vi "SigProc_subVI smoothBoxcarAvg.vi"(6 "Size":i32=1 min=1 max=100000, 11 "Spectra in":cluster{"X":dbl[], "Y":dbl[]}[](array[cluster])) -> (3 "Spectra out":cluster{"X":dbl[], "Y":dbl[]}[](array[cluster]))   [LabVIEW 2018, in "Sig2MS.lvclass"]
uses:
  Sig2MS.lvclass
  <vilib>/Analysis/baseanly.llb/Mean (DBL).vi
  <vilib>/Analysis/NI_AALBase.lvlib
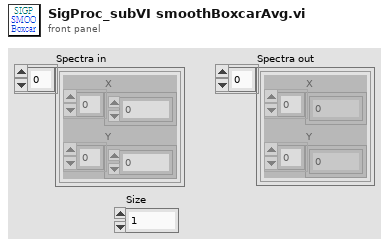
[diagram p1: front panel]
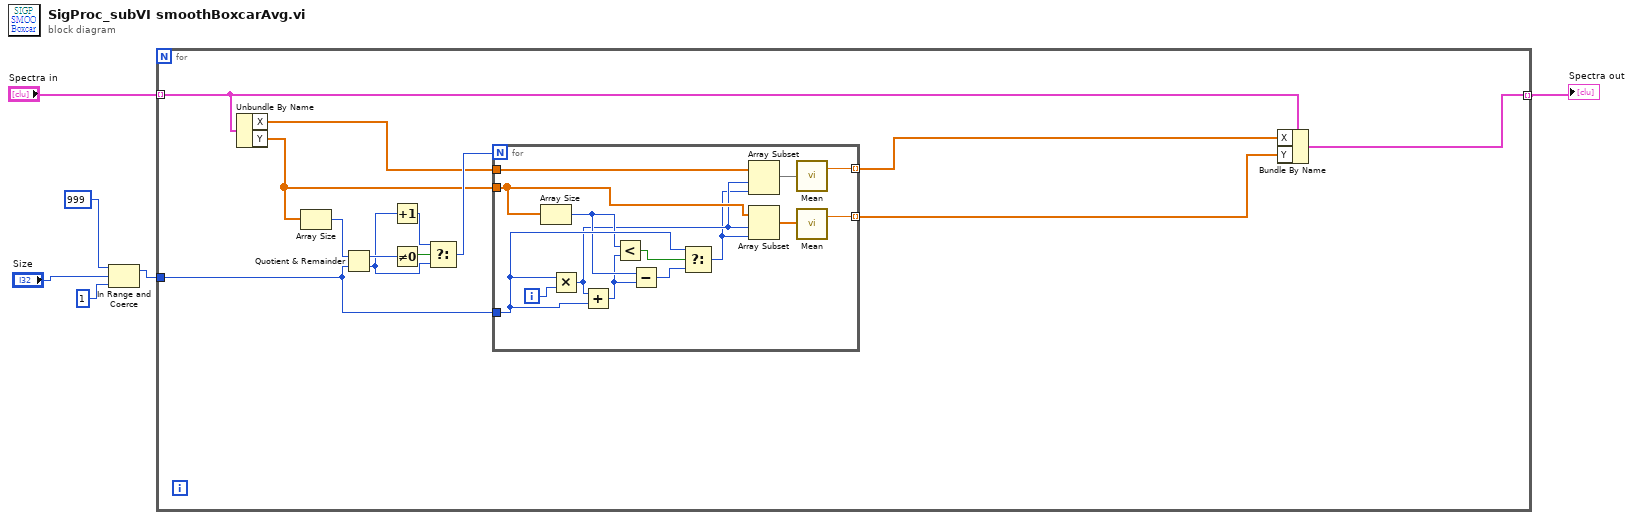
[diagram p0: block diagram]
diagram:
  n1 = In Range and Coerce(upper limit=999, x="Size", lower limit=1) -> (coerced(x)=w1:i32)  [unwired: 1 out]
  n2 = for {
    tunnel: "Spectra in" -> [w19] mode=indexing
    tunnel: [w18] -> w6 mode=indexing
    tunnel: w1 -> [w17]
    n3 = Unbundle By Name(w19) -> ("X"=w10:dbl[], "Y"=w9:dbl[])
    n4 = Array Size(array=w9) -> (size(s)=w16:i32)
    n5 = Quotient & Remainder(x=w16, y=w17) -> (x-y*floor(x/y)=w15:i32, floor(x/y)=w12:i32)
    n6 = Increment(x=w12) -> (x+1=w13:i32)
    n7 = Not Equal To 0?(x=w15) -> (x != 0?=w14:bool)
    n8 = Select(t=w13, s=w14, f=w12) -> (s? t:f=w11:i32)
    n9 = for {
      N: w11 -> [_]
      tunnel: w10 -> [w26]
      tunnel: w9 -> [w27]
      tunnel: w17 -> [w31]
      tunnel: [w21] -> w7 mode=indexing
      tunnel: [w20] -> w8 mode=indexing
      i -> [w33]
      n10 = Array Size(array=w27) -> (size(s)=w30:i32)
      n11 = Multiply(x=w31, y=w33) -> (x*y=w25:i32)
      n12 = Add(x=w25, y=w31) -> (x+y=w29:i32)
      n13 = Less?(x=w30, y=w29) -> (x < y?=w32:bool)
      n14 = Subtract(x=w30, y=w29) -> (x-y=w28:i32)
      n15 = Select(t=w31, s=w32, f=w28) -> (s? t:f=w24:i32)
      n16 = Array Subset(array=w26, index=w25, length=w24) -> (w23:dbl[])
      n17 = Array Subset(array=w27, index=w25, length=w24) -> (w22:dbl[])
      n18 = call-poly <vilib>:"Mean.vi"("X"=w23) -> ("mean"=w21:dbl)  [unwired: 1 out]
      n19 = call-poly <vilib>:"Mean.vi"("X"=w22) -> ("mean"=w20:dbl)  [unwired: 1 out]
    }
    n20 = Bundle By Name(cluster=w19, "X"=w7, "Y"=w8) -> (w18:cluster{"X":dbl[], "Y":dbl[]})
  }
  "Spectra out" <- w6
